vi "CTRE_PigeonIMU_SetYaw.vi"(8 "error in (no error)":errorcluster, 9 "TareType (SetValue)":T1 items=["SetValue"=0, "AddOffset"=1, "MatchCompass"=2, "SetOffset"=255], 10 "Value":dbl, 11 "PigeonIMUDevRef":T2={"DeviceStatus"={"status"=FALSE, "code"=0, "source"=""}, "Device Number"=0, "Type"=352321536, "Device ID"=0} {"Type" items=["CAN"=352321536, "TalonSRX"=33554432]}) -> (0 "error out":errorcluster, 3 "PigeonIMUDevRef":T2={"DeviceStatus"={"status"=FALSE, "code"=0, "source"=""}, "Device Number"=0, "Type"=352321536, "Device ID"=0} {"Type" items=["CAN"=352321536, "TalonSRX"=33554432]})   [LabVIEW 2016]
uses:
  <vilib>/Rock Robotics/WPI/ThirdParty/Sensors/Pigeon IMU/CTRE_PigeonIMU_DeviceRef.ctl
  <vilib>/Rock Robotics/WPI/ThirdParty/Sensors/Pigeon IMU/CTRE_PigeonIMU_ConnectionType.ctl
  <vilib>/Rock Robotics/WPI/ThirdParty/Sensors/Pigeon IMU/CTRE_PigeonIMU_TareType.ctl
  <vilib>/Rock Robotics/WPI/ThirdParty/Sensors/Pigeon IMU/CTRE_PigeonIMU_Params.ctl
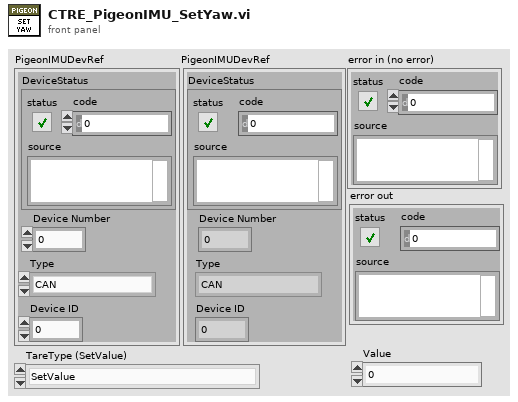
[diagram p1: front panel]
types:
  T1 = typedef "CTRE_PigeonIMU_TareType.ctl" = u8
  T2 = typedef "CTRE_PigeonIMU_DeviceRef.ctl" = cluster{"DeviceStatus":errorcluster, "Device Number":u8, "Type":T3, "Device ID":u32}
  T3 = typedef "CTRE_PigeonIMU_ConnectionType.ctl" = u32
  T4 = typedef "CTRE_PigeonIMU_Params.ctl" = u8
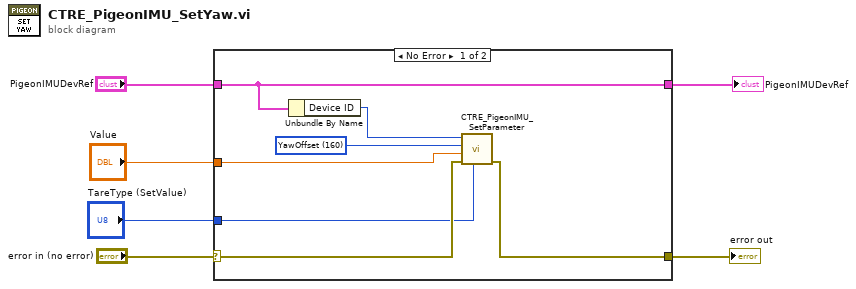
[diagram p0: block diagram]
diagram:
  n1 = case shown="No Error" "error in (no error)" {
    selector: "error in (no error)" -> [w9 w14]
    tunnel: [w8 w14] -> w5
    tunnel: [w13 w15] -> w3
    tunnel: "PigeonIMUDevRef" -> [w13 w15]
    tunnel: "Value" -> [w10 _]
    tunnel: "TareType (SetValue)" -> [w7 _]
    frame No Error {
      w11 = T4 160 items=["YawOffset"=160, "CompassOffset"=161, "BetaGain"=162, "Reserved163"=163, "GyroNoMotionCal"=164, "EnterCalibration"=165, "FusedHeadingOffset"=166] ("Parameter")
      n2 = Unbundle By Name(w13) -> ("Device ID"=w12:u32)
      n3 = call <vilib>:"CTRE_PigeonIMU_SetParameter.vi"("TareType"=w7, "error in (no error)"=w9, "Value"=w10, "Parameter"=w11, "Device ID (0)"=w12) -> ("error out"=w8:errorcluster)  [unwired: 5 in, 1 out]
    }
    frame Error {
    }
  }
  "PigeonIMUDevRef" <- w3
  "error out" <- w5
